vi "readIMU.vi"(2 "Address":u8 format="%x", 3 "Frames to Read":u8, 4 "SPI Config In":T1) -> (0 "Data Read":u8[](array[numeric]) format="%x", 1 "SPI Config Out":T1)   [LabVIEW 2019]
uses:
  SPI/SPI Config.ctl
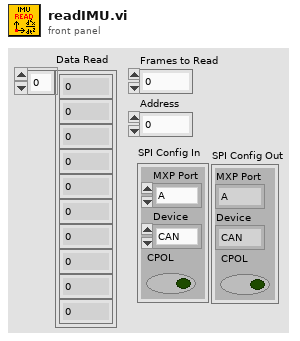
[diagram p1: front panel]
types:
  T1 = typedef "SPI Config.ctl" = cluster{"MXP Port":enum16{"A", "B"}, "Device":enum16{"CAN", "ENC", "IMU1", "IMU2"}, "CPOL":bool}
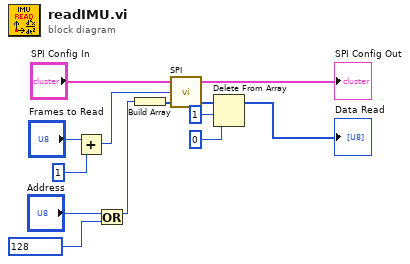
[diagram p0: block diagram]
diagram:
  n1 = Add(x="Frames to Read", y=u8 1) -> (x+y=w10:u8)
  n2 = Or(x="Address", y=u8 128) -> (x .or. y?=w6:u8)
  n3 = Build Array(w6) -> (w8:u8[])
  n4 = call "SPI.vi"("Data to Write"=w8, "Frames to Write"=w10, "SPI Config In"="SPI Config In") -> ("Data Read"=w4:u8[], "SPI Config Out"=→"SPI Config Out":T1)  [unwired: 1 out]
  n5 = Delete From Array(array=w4, length=1, index=0) -> (array with subset deleted=→"Data Read":u8[])  [unwired: 1 out]
